vi "Telescope Convert HHMMSS string.vi"(10 "RA String":string) -> (2 "Right Ascension":T1)   [LabVIEW 2024, in "Telescope.lvclass"]
uses:
  Telescope.lvclass
  Telescope cluster Dec.ctl
  <vilib>/regexp/Match Regular Expression.xnode
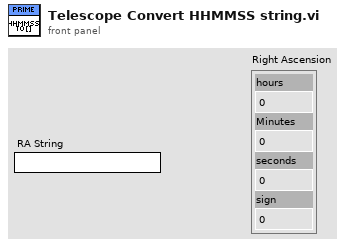
[diagram p1: front panel]
types:
  T1 = typedef "Telescope cluster Dec.ctl" = cluster{"hours":dbl, "Minutes":dbl, "seconds":dbl, "sign":dbl}
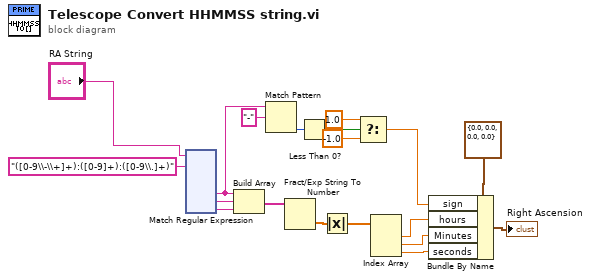
[diagram p0: block diagram]
diagram:
  n1 = xnode "Match Regular Expression"("input string"="RA String", "regular expression"="([0-9\\-\\+]+):([0-9]+):([0-9\\.]+)") -> ("submatch 1"=w14:string, "submatch 2"=w18:string, "submatch 3"=w17:string)  [unwired: 4 in, 5 out]
  n2 = Build Array(w14, w18, w17) -> (w16:string[])
  n3 = Match Pattern(string=w14, regular expression="-") -> (offset past match=w12:i32)  [unwired: 1 in, 3 out]
  n4 = Fract/Exp String To Number(string=w16) -> (number=w11:dbl[])  [unwired: 3 in, 1 out]
  n5 = Less Than 0?(x=w12) -> (x < 0?=w8:bool)
  n6 = Absolute Value(x=w11) -> (abs(x)=w10:dbl[])
  n7 = Select(t=1.0, s=w8, f=-1.0) -> (s? t:f=w5:dbl)
  n8 = Index Array(array=w10) -> (element #1=w4:dbl, element #2=w3:dbl, element #3=w2:dbl)  [unwired: 3 in]
  n9 = Bundle By Name(cluster=T1 {"hours"=0.0, "Minutes"=0.0, "seconds"=0.0, "sign"=0.0} ("Right Ascension"), "sign"=w5, "hours"=w4, "Minutes"=w3, "seconds"=w2) -> (→"Right Ascension":T1)
